vi "Choreo_TrajectoryDifferential_Samples.vi"(11 "ChoreoTrajectoryDifferential":T2) -> (3 "samples":T1[](array[typedef]))   [LabVIEW 2019, in "ChoreoLib.lvlib"]
doc: "Returns the samples of the trajectory.\n \nInputs:\n -- ChoreoTrajectorySwerve - cluster - data cluster for this trajectory \n\nOutputs: \n -- samples - SwerveSample - the samples of the trajectory."
uses:
  TypeDef/ChoreoEventMarker.ctl
  ChoreoLib.lvlib
  TypeDef/ChoreoDifferentialSample.ctl
  TypeDef/ChoreoTrajectoryDifferential.ctl
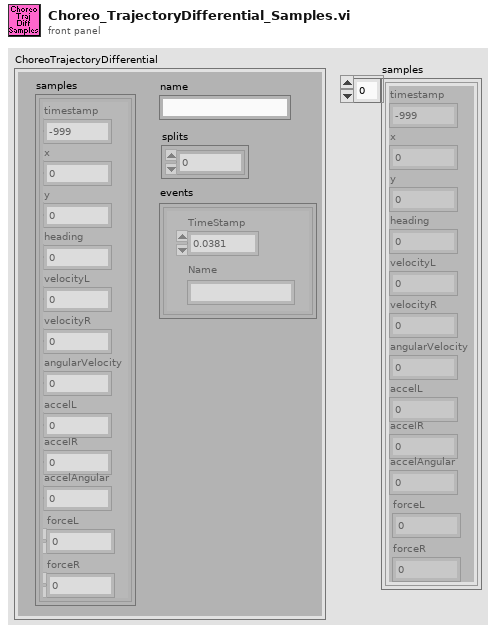
[diagram p1: front panel]
types:
  T1 = typedef "ChoreoLib.lvlib/ChoreoDifferentialSample.ctl" = cluster{"timestamp":dbl, "x":dbl, "y":dbl, "heading":dbl, "velocityL":dbl, "velocityR":dbl, "angularVelocity":dbl, "accelL":dbl, "accelR":dbl, "accelAngular":dbl, "forceL":dbl, "forceR":dbl}
  T2 = typedef "ChoreoLib.lvlib/ChoreoTrajectoryDifferential.ctl" = cluster{"name":string, "samples":T1[], "splits":i32[], "events":T3[]}
  T3 = typedef "ChoreoLib.lvlib/ChoreoEventMarker.ctl" = cluster{"TimeStamp":dbl, "Name":string}
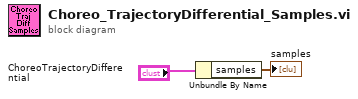
[diagram p0: block diagram]
diagram:
  n1 = Unbundle By Name("ChoreoTrajectoryDifferential") -> ("samples"=→"samples":T1[])
